vi "UpConvert - 1ch.vi"(5 "clock x2":refnum<k21>="Daughterboard 0\\Data Clock x2", 7 "reset":bool, 8 "input valid":bool, 10 "output sample rate":fxp<+,48,1>, 11 "data in":T1=[{"I"=0.0, "Q"=0.0, "overflow"=FALSE}]) -> (0 "output valid":bool, 3 "data out":T1)   [LabVIEW 2025]
uses:
  IQ-1element.ctl
  <instrlib>/_niInstr/DSP/v1/Shared/Public/IQ Data.ctl
  <instrlib>/_niInstr/DSP/v1/FPGA/niInstr DSP v1 FPGA.lvlib
  <instrlib>/_niInstr/DSP/v1/Shared/niInstr DSP v1 Shared.lvlib
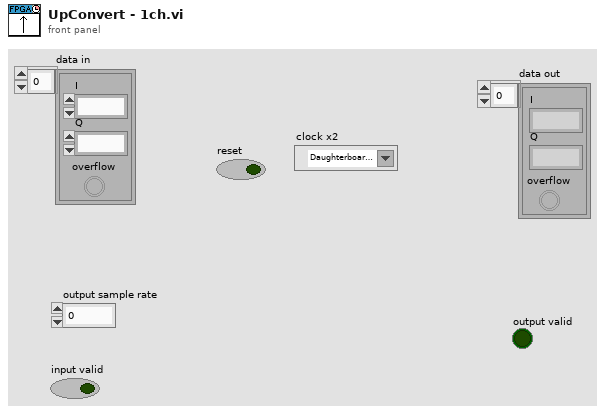
[diagram p1: front panel]
types:
  T1 = typedef "IQ-1element.ctl" = T2[]
  T2 = typedef "niInstr DSP v1 Shared.lvlib/IQ Data.ctl" = cluster{"I":fxp<+/-,18,1>, "Q":fxp<+/-,18,1>, "overflow":bool}
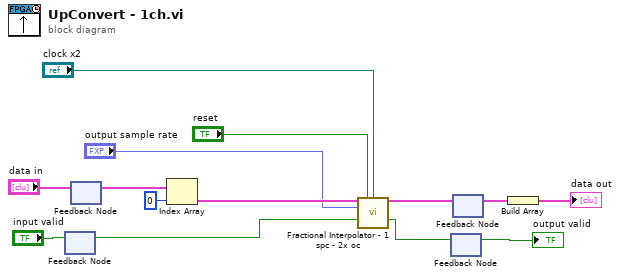
[diagram p0: block diagram]
diagram:
  n1 = feedback #1() -> (w4:bool)  [unwired: 1 in]
  n2 = feedback-in #1("input valid") -> ()
  n3 = feedback #2() -> (w5:T1)  [unwired: 1 in]
  n4 = feedback-in #2("data in") -> ()
  n5 = Index Array(array=w5, index=0) -> (element=w12:T2)
  n6 = call <instrlib>:"Fractional Interpolator - 1 spc - 2x oc.vi"("data in"=w12, "reset"="reset", "clock x 2"="clock x2", "input sample rate"="output sample rate", "input valid"=w4) -> ("data out"=w11:T2, "output valid"=w3:bool)  [unwired: 7 in, 2 out]
  n7 = feedback #3() -> (→"output valid":bool)  [unwired: 1 in]
  n8 = feedback-in #3(w3) -> ()
  n9 = feedback #4() -> (w13:T2)  [unwired: 1 in]
  n10 = feedback-in #4(w11) -> ()
  n11 = Build Array(w13) -> (→"data out":T2[])
